vi "Byte Buffer.Get Buffer String.vi"(7 "offset (0)":u64, 8 "error in (no error)":errorcluster, 9 "length (-1: rest)":i64=-1, 10 "allocated string in":string, 11 "Byte Buffer in":refnum<class "Byte Buffer.lvclass">) -> (0 "error out":errorcluster, 2 "string out":string, 3 "Byte Buffer out":refnum<class "Byte Buffer.lvclass">)   [LabVIEW 2016, in "VeriStand Data.lvlib" / "Byte Buffer.lvclass"]
uses:
  Byte Buffer.lvclass
  Byte Buffer.lvclass/Byte Buffer.ctl
  Memory Management/Memory Management.Handle Return.vi
  VeriStand Data.lvlib
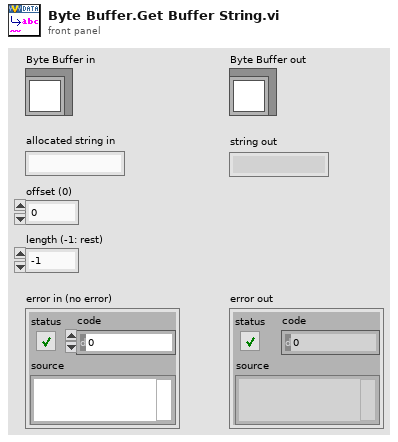
[diagram p1: front panel]
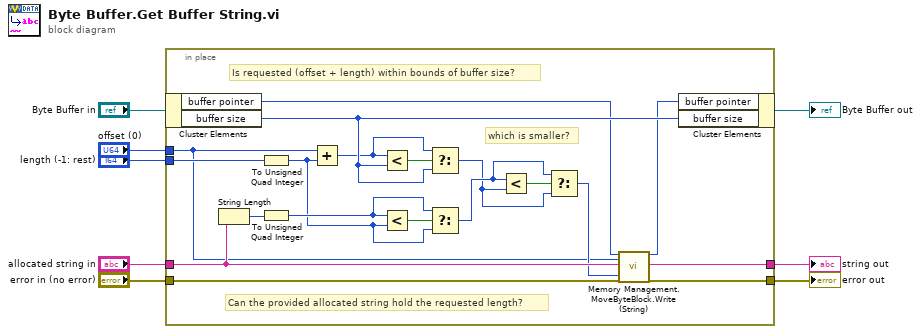
[diagram p0: block diagram]
diagram:
  n1 = in-place {
    in-place-border: "error in (no error)" -> [w26]
    in-place-border: "allocated string in" -> [w23]
    in-place-border: "length (-1: rest)" -> [w20]
    in-place-border: "offset (0)" -> [w10]
    in-place-border: [w19] -> w3
    in-place-border: [w18] -> w2
    # "which is smaller?"
    # "Can the provided allocated string hold the requested length?"
    # "Is requested (offset + length) within bounds of buffer size?"
    n2 = in-place-cluster #1("Byte Buffer in") -> ("buffer pointer"=w22:u64, "buffer size"=w27:u64)
    n3 = String Length(string=w23) -> (length=w24:i32)
    n4 = To Unsigned Quad Integer(1:w20) -> (0:w15:u64)
    n5 = To Unsigned Quad Integer(1:w24) -> (0:w16:u64)
    n6 = Add(x=w10, y=w15) -> (x+y=w21:u64)
    n7 = Less?(x=w21, y=w27) -> (x < y?=w25:bool)
    n8 = Less?(x=w16, y=w15) -> (x < y?=w17:bool)
    n9 = Select(t=w21, s=w25, f=w27) -> (s? t:f=w12:u64)
    n10 = Select(t=w16, s=w17, f=w15) -> (s? t:f=w13:u64)
    n11 = Less?(x=w13, y=w12) -> (x < y?=w14:bool)
    n12 = Select(t=w13, s=w14, f=w12) -> (s? t:f=w11:u64)
    n13 = call "Memory Management.MoveByteBlock.Write (String).vi"("src ptr in"=w22, "src offset (0)"=w10, "dst in"=w23, "size"=w11, "error in (no error)"=w26) -> ("src ptr out"=w9:u64, "dst out"=w18:string, "error out"=w19:errorcluster)  [unwired: 9 in, 3 out]
    n14 = in-place-cluster #1("buffer pointer"=w9, "buffer size"=w27) -> (→"Byte Buffer out":refnum<class "Byte Buffer.lvclass">)
  }
  "error out" <- w3
  "string out" <- w2
